vi "Start.vi"(8 "Error In":errorcluster, 11 "reference in":refnum<class "Instrument.lvclass">) -> (0 "Error Out":errorcluster, 3 "reference out":refnum<class "Instrument.lvclass">)   [LabVIEW 2024, in "HAL.lvlib" / "Instrument.lvclass"]
uses:
  Instrument.lvclass
  Configurations/CFG Base/CFG Base.lvclass
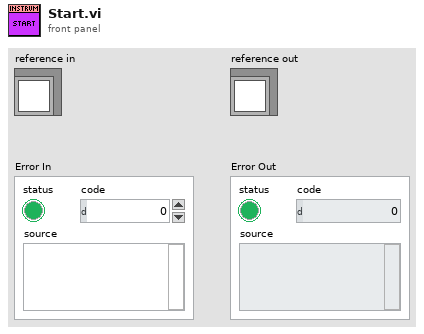
[diagram p1: front panel]
types:
  T1 = typedef "HAL.lvlib/Instrument.lvclass/ObjectAttributes.ctl" = cluster{"CFG Base":refnum<class "CFG Base.lvclass">, "Started Counter":i16}
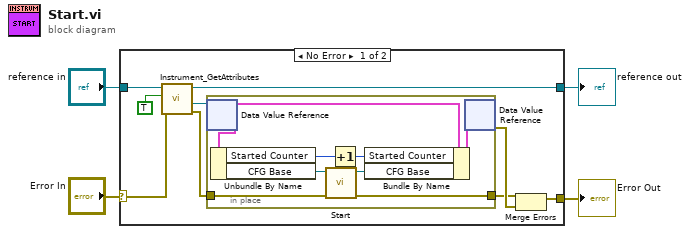
[diagram p0: block diagram]
diagram:
  n1 = case shown="No Error" "Error In" {
    selector: "Error In" -> [w12 w23]
    tunnel: [w9 w23] -> w3
    tunnel: [w10 w22] -> w1
    tunnel: "reference in" -> [w13 w22]
    frame No Error {
      n2 = call "Instrument_GetAttributes.vi"("Error In"=w12, "OnlyGetDvrReference(False)"=TRUE, "reference in"=w13) -> ("Error Out"=w6:errorcluster, "DataRef"=w8:refnum<data-value>, "reference out"=w10:refnum<class "Instrument.lvclass">)  [unwired: 5 in, 1 out]
      n3 = in-place {
        in-place-border: w6 -> [w17]
        in-place-border: [w16] -> w5
        n4 = in-place-dvr #1(w8) -> (w20:T1)  [unwired: 1 out]
        n5 = Unbundle By Name(w20) -> ("Started Counter"=w15:i16, "CFG Base"=w18:refnum<class "CFG Base.lvclass">)
        n6 = call-dynamic "Start.vi"("error in"=w17, "CFG Base in"=w18) -> ("error out"=w16:errorcluster, "CFG Base out"=w19:refnum<class "CFG Base.lvclass">)  [unwired: 8 in]
        n7 = Increment(x=w15) -> (x+1=w14:i16)
        n8 = Bundle By Name(cluster=w20, "Started Counter"=w14, "CFG Base"=w19) -> (w21:T1)
        n9 = in-place-dvr #1(w21) -> (w11:errorcluster)  [unwired: 1 out]
      }
      n10 = Merge Errors(w5, w11) -> (w9:errorcluster)
    }
    frame Error {
    }
  }
  "Error Out" <- w3
  "reference out" <- w1
